vi "Disconnect with server.vi"(8 "error in (no error)":errorcluster, 11 "Control-Client in":refnum<class "Control-Client.lvclass">) -> (0 "error out":errorcluster, 3 "Control-Client out":refnum<class "Control-Client.lvclass">)   [LabVIEW 2020, in "Control-Client.lvclass"]
uses:
  Control-Client.lvclass
  C:/dev/TRANCON/Classes/GeneralFunctionality/GeneralFunctionality.lvclass
  <vilib>/NI/STM/TCP/TCP Connection Info.ctl
  <vilib>/NI/STM/SubVIs/MetaDataElement.ctl
  Control-Client.lvclass/Control-Client.ctl
  dependecies/ControlsVIs/Clusters-def/Message types.ctl
  dependecies/ControlsVIs/Clusters-def/Commands-CLIENT.ctl
  <vilib>/NI/STM/NI STM.lvlib
  Message/Message.lvclass
  GeneralFunctionality/GeneralFunctionality.lvclass
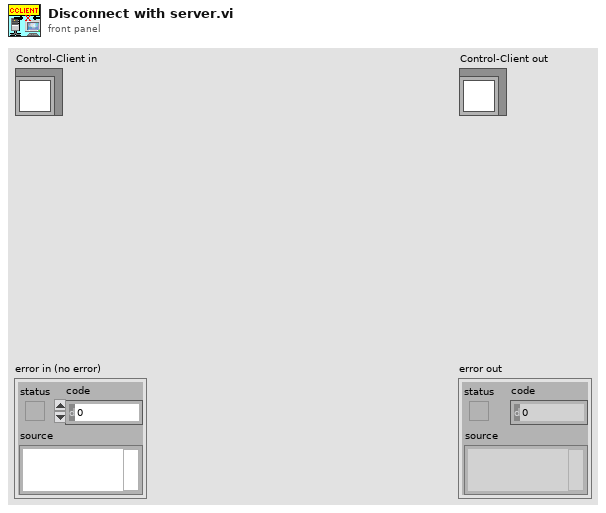
[diagram p1: front panel]
types:
  T1 = typedef "NI STM.lvlib/TCP Connection Info.ctl" = cluster{"connection ID":refnum<k5>, "meta data":T2[]}
  T2 = typedef "NI STM.lvlib/MetaDataElement.ctl" = string
  T3 = typedef "Control-Client.lvclass/Commands-CLIENT.ctl" = string
  T4 = typedef "Message types.ctl" = string
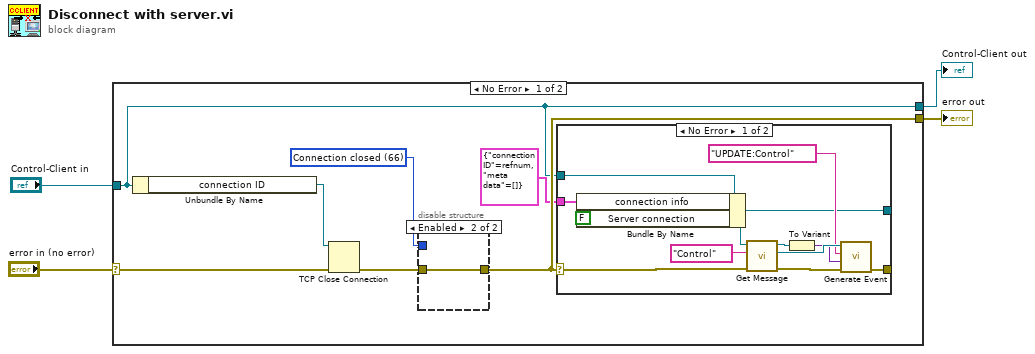
[diagram p0: block diagram]
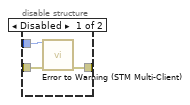
[diagram p2: hidden frame]
diagram:
  n1 = case shown="No Error" "error in (no error)" {
    selector: "error in (no error)" -> [w8 w31]
    tunnel: [w7 w31] -> w3
    tunnel: [w6 w30] -> w1
    tunnel: "Control-Client in" -> [w6 w30]
    frame No Error {
      w10 = 66 items=["No Error", "Argument Error", "Memory Full", "Out of Zone", "End of File", "File Already Open", "Generic File IO Error", "File Not Found", "File Permission Error", "Disk Full", "Duplicate Path", "Too Many Files Open", "Not Enabled", "Resource File Not Found", "Cannot Add Resource", "Resource Not Found", "Image Not Found", "Image Memory Error", "Pen Does Not Exist", "Config Bad Type", "Config Token Not Found", "Config Parse Error", "Config Memory Error", "Bad External Code Format", "Bad External Code Offset", "External Code Not Present", "Null Window", "Destroy Window Mixup", "Null Menu", "Print Aborted", "Bad Print Record", "Print Driver Error", "Windows Error During Print", "Memory Error During Print", "Print Dialog Error", "Generic Print Error", "Invalid Device Refnum", "Device Not Found", "Device Parameter Error", "Device Unit Error", "Can't Open Device", "Device Call Aborted", "Generic Error", "Cancelled By User", "Object ID Too Low", "Object ID Too High", "Object Not In Heap", "Unknown Heap", "Bad DefProc ID", "DefProc Not In Table", "Message Out Of Range", "Null Method", "Unknown Message", "Manager Call Not Supported", "Bad address", "Connection In progress", "Connection timed out", "Connection is already in progress", "Network attribute not supported", "Network error", "Address in use", "System out of memory", "Connection aborted", "Connection refused", "Connection is not connected", "Connection is already connected", "Connection closed", "Initialize error (interapplication manager)", "Bad occurrence", "Wait on unbound occurrence handler", "Occurrence queue overflow", "Bad path", "Semaphore not signaled", "Unrecognized type (interapplication manager)"] ("1st Error to Convert")
      n2 = Unbundle By Name(w6) -> ("connection ID"=w11:refnum<k5>)
      n3 = TCP Close Connection(connection ID=w11, error in (no error)=w8) -> (error out=w9:errorcluster)  [unwired: 1 in, 1 out]
      n4 = disable-structure shown="Enabled" {
        disable-tunnel: w10 -> [w14 _]
        disable-tunnel: w9 -> [w13 w15]
        disable-tunnel: [w12 w15] -> w7
        frame Disabled {
          n5 = call "Error to Warning (STM Multi-Client).vi"("1st Error to Convert"=w14, "error in"=w13) -> ("warning out"=w12:errorcluster)  [unwired: 13 in]
        }
        frame Enabled {
        }
      }
      n6 = case shown="No Error" w7 {
        selector: w7 -> [w17 w28]
        tunnel: w6 -> [w27 w29]
        tunnel: [w18 w29] -> _
        tunnel: T1 {"connection ID"=refnum, "meta data"=[]} ("connection info") -> [w26 _]
        tunnel: [w16 w28] -> _
        frame No Error {
          n7 = Bundle By Name(cluster=w27, "connection info"=w26, "Server connection"=FALSE) -> (w18:refnum<class "Control-Client.lvclass">)
          n8 = call "Get Message.vi"("error in (no error)"=w17, "Message type"=T4 "Control", "GeneralFunctionality en entrée"=w18) -> ("error out"=w22:errorcluster, "Message.lvclass"=w21:refnum<class "Message.lvclass">, "GeneralFunctionality en sortie"=w24:refnum<class "Control-Client.lvclass">)  [unwired: 6 in]
          n9 = To Variant(anything=w24) -> (Variant=w19:variant)
          n10 = call "Generate Event.vi"("error in (no error)"=w22, "Data"=w19, "Command"=T3 "UPDATE:Control" ("Commands-Client"), "Message en entrée"=w21) -> ("error out"=w16:errorcluster)  [unwired: 6 in, 1 out]
        }
        frame Error {
        }
      }
    }
    frame Error {
    }
  }
  "error out" <- w3
  "Control-Client out" <- w1
